vi "Lab0_Visibility.vi"() -> ()   [LabVIEW 2014]
panel:
  in  "stop":bool
  in  "Click to toggle string":bool
  out "String":string
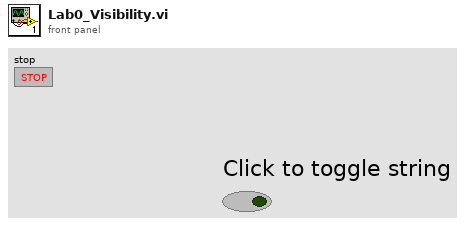
[diagram p1: front panel]
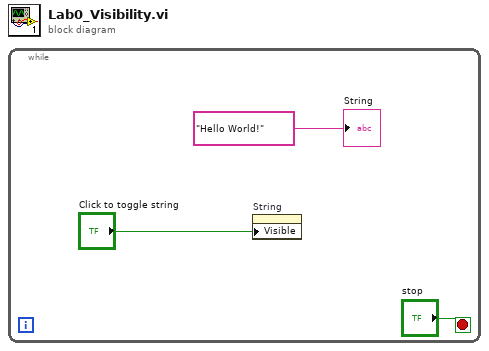
[diagram p0: block diagram]
diagram:
  n1 = while {
    stop <- "stop" stop-if-true
    n2 = property on="String" class="Str"("Visible"="Click to toggle string") -> ()  [unwired: 2 in, 2 out]
    "String" <- "Hello World!"
  }
